vi "pump_01.vi"() -> ()   [LabVIEW 2018]
panel:
  in  "time for move (ms)":u32=1000
  in  "rate (ml/min)":dbl=0.001
  in  "VISA resource name":refnum<visa-resource-name>="COM3"
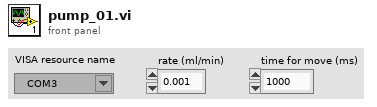
[diagram p1: front panel]
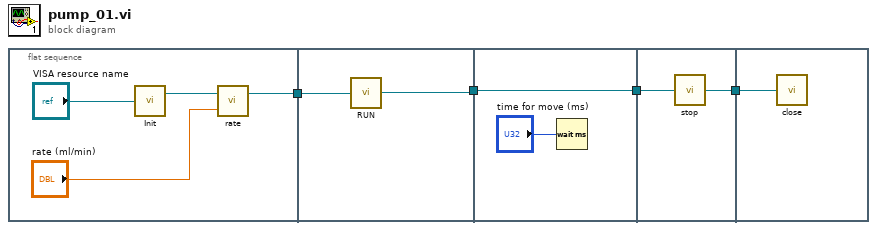
[diagram p0: block diagram]
diagram:
  n1 = flat-sequence {
    tunnel: [w5] -> w4
    tunnel: w4 -> [w9]
    tunnel: [w10] -> w3
    tunnel: [w11] -> w2
    tunnel: w3 -> [w11]
    tunnel: w2 -> [w14]
    tunnel: [w13] -> w1
    tunnel: w1 -> [w15]
    frame #0 {
      n2 = call <instrlib>:"Init.vi"("VISA resource name"="VISA resource name") -> ("VISA resource name out"=w7:refnum<visa-resource-name>)  [unwired: 1 out]
      n3 = call <instrlib>:"rate.vi"("rate"="rate (ml/min)", "VISA resource name"=w7) -> ("VISA resource name out"=w5:refnum<visa-resource-name>)  [unwired: 1 out]
    }
    frame #1 {
      n4 = call <instrlib>:"RUN.vi"("VISA resource name"=w9) -> ("VISA resource name out"=w10:refnum<visa-resource-name>)  [unwired: 1 out]
    }
    frame #2 {
      n5 = Wait (ms)(milliseconds to wait="time for move (ms)") -> ()  [unwired: 1 out]
    }
    frame #3 {
      n6 = call <instrlib>:"stop.vi"("VISA resource name"=w14) -> ("VISA resource name out"=w13:refnum<visa-resource-name>)
    }
    frame #4 {
      n7 = call <instrlib>:"close.vi"("VISA resource name"=w15) -> ()
    }
  }
